vi "Cross_spectra_Display.vi"(4 "U1 U2 phase":cluster{dbl, dbl, dbl[]}(graph), 5 "U1 U2 coherence":cluster{dbl, dbl, dbl[]}(graph), 6 "U2 spectra":cluster{dbl, dbl, dbl[]}(graph), 7 "U1 spectra":cluster{dbl, dbl, dbl[]}(graph)) -> ()   [LabVIEW 2010]
panel:
  in  "Velocity arrays":dbl[][](array[numeric]) format="%.2f"
  in  "Sampling Rate (Hz)":sgl=1000.0 min=0 format="%.2f"
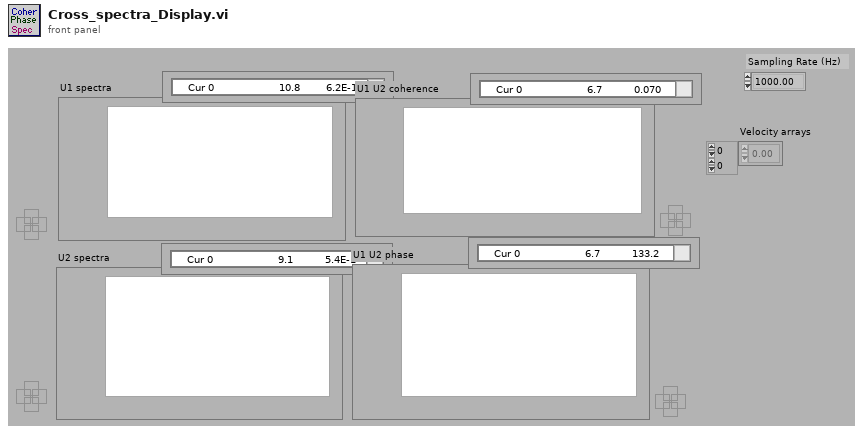
[diagram p1: front panel]
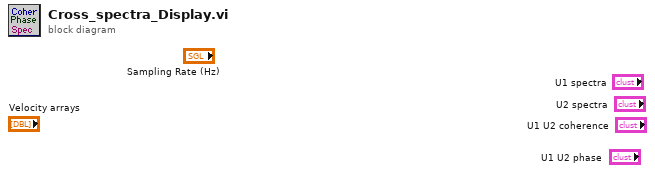
[diagram p0: block diagram]
diagram:
